vi "Tree Test-1.vi"() -> ()   [LabVIEW 2015]
panel:
  out "Numeric2":i32
  out "Stop 2":bool
  in  "number":i32
  out "Single Selection Display Text":string
  in  "Single Selection Tree":string(tree)="Sine Graph"
  in  "Stop":bool
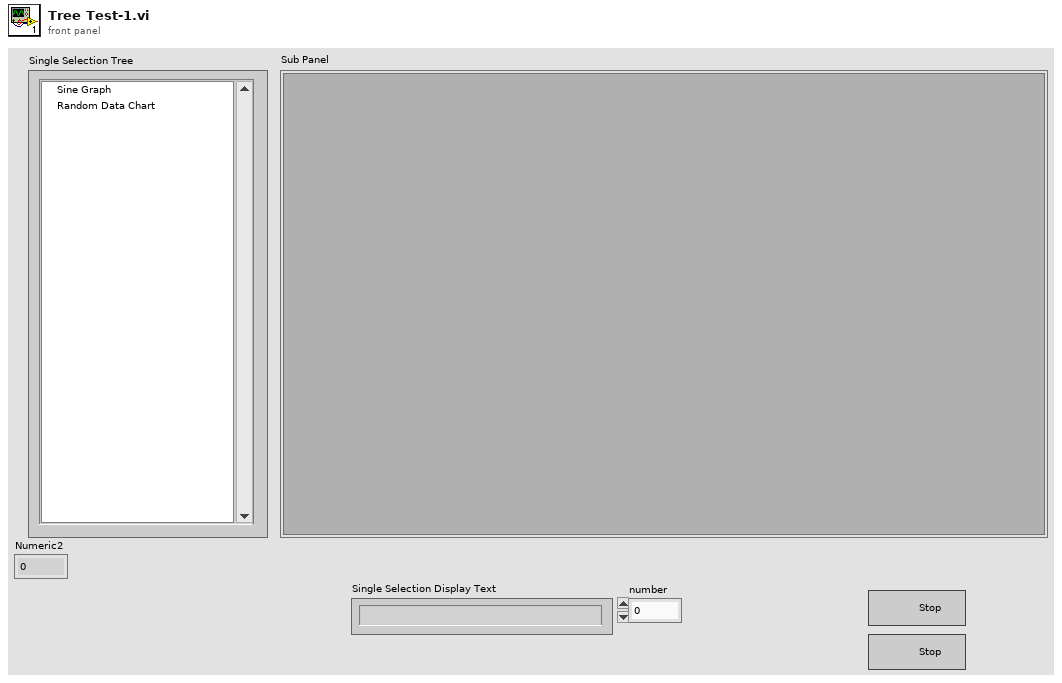
[diagram p1: front panel]
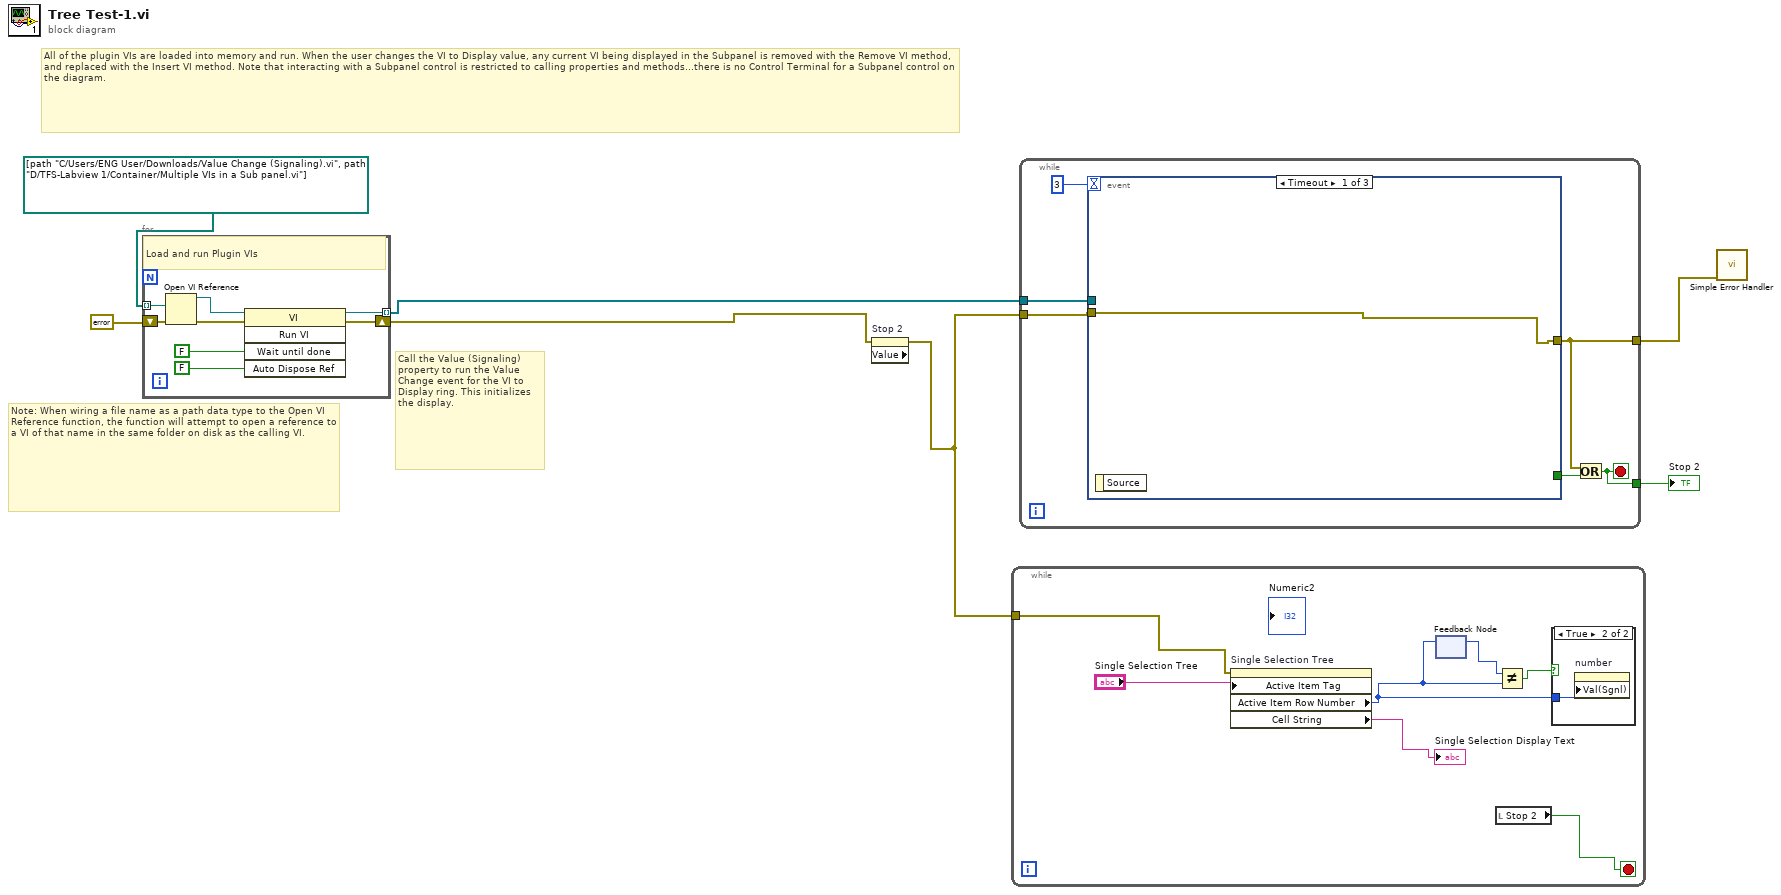
[diagram p0: block diagram]
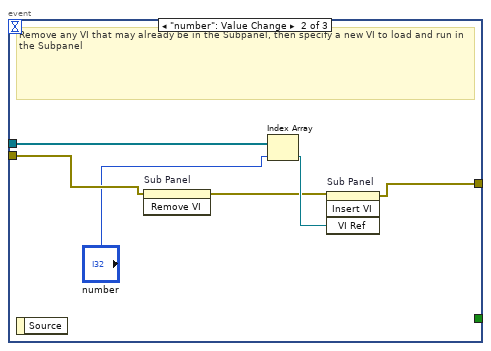
[diagram p3: hidden frame]
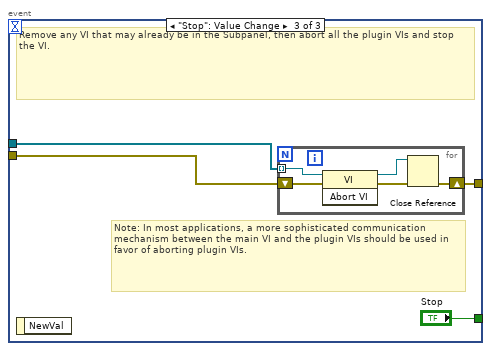
[diagram p4: hidden frame]
diagram:
  # "All of the plugin VIs are loaded into memory and run. When the user changes the VI to Display value, any current VI being displayed in the Subpanel is removed with the Remove VI method, and replaced with the Insert VI method. Note that interacting with a Subpanel control is restricted to calling properties and methods...there is no Control Terminal for a Subpanel control on the diagram."
  # "Note: When wiring a file name as a path data type to the Open VI Reference function, the function will attempt to open a reference to a VI of that name in the same folder on disk as the calling VI."
  # "Call the Value (Signaling) property to run the Value Change event for the VI to Display ring. This initializes the display."
  n1 = for {
    tunnel: path[] [path "C:/Users/ENG User/Downloads/Value Change (Signaling).vi", path "D:/TFS-Labview 1/Container/Multiple VIs in a Sub panel.vi"] -> [w11] mode=indexing
    tunnel: [w10] -> w6 mode=indexing
    shift-right: [w8] -> w2
    shift-left: errorcluster {"status"=FALSE, "code"=0, "source"=""} ("error constant") -> [w9]
    # "Load and run Plugin VIs"
    n2 = Open VI Reference(vi path=w11, error in (no error)=w9) -> (vi reference=w12:refnum<vi>, error out=w13:errorcluster)  [unwired: 4 in]
    n3 = invoke class="VI" method="Run VI"(reference=w12, error in=w13, "Wait until done"=FALSE ("Wait Until Done"), "Auto Dispose Ref"=FALSE ("Auto Dispose Reference")) -> (reference out=w10:refnum<vi>, error out=w8:errorcluster)  [unwired: 1 in, 3 out]
  }
  n4 = property on="Stop 2" class="Bool" props=["Value"](error in=w2) -> (error out=w1:errorcluster)  [unwired: 1 in, 2 out]
  n5 = while {
    tunnel: w1 -> [w19]
    stop <- w20 stop-if-true
    n6 = property on="Single Selection Tree" class="TreeControl (strict)"(error in=w19, "Active Item Tag"="Single Selection Tree") -> ("Active Item Row Number"=w17:i32, "Cell String"=→"Single Selection Display Text":string)  [unwired: 1 in, 2 out]
    n7 = feedback-in #1(w17) -> ()
    n8 = feedback #1() -> (w18:i32)  [unwired: 1 in]
    n9 = local read "Stop 2"() -> (w20:bool)
    n10 = Not Equal?(x=w18, y=w17) -> (x != y?=w16:bool)
    n11 = case shown="True" w16 {
      tunnel: w17 -> [_ w23]
      frame False {
      }
      frame True {
        n12 = property on="number" class="DigNum (strict)"("Val(Sgnl)"=w23) -> ()  [unwired: 2 in, 2 out]
      }
    }
  }
  n13 = while {
    tunnel: [w28] -> w7
    tunnel: w6 -> [w24]
    tunnel: w1 -> [w25]
    tunnel: [w26] -> w3
    stop <- w26 stop-if-true
    n14 = event shown="[0] Timeout" {
      selector: _ -> [_ _ _]
      dyn-events: _ -> [_ _ _]
      timeout: 3 -> [_ _ _]
      tunnel: [_ _ "Stop"] -> w29
      tunnel: [w30 w34 w38] -> w28
      tunnel: w24 -> [_ w36 w39]
      tunnel: w25 -> [w30 w32 w37]
      event Timeout {
        n15 = event-data() -> ()  [unwired: 1 in, 1 out]
      }
      event "number": Value Change {
        # "Remove any VI that may already be in the Subpanel, then specify a new VI to load and run in the Subpanel"
        n16 = event-data() -> ()  [unwired: 1 in, 1 out]
        n17 = invoke on="Sub Panel" class="SubPnl" method="Remove VI"(error in=w32) -> (error out=w33:errorcluster)  [unwired: 2 in, 2 out]
        n18 = Index Array(array=w36, index="number") -> (element=w35:refnum<vi>)
        n19 = invoke on="Sub Panel" class="SubPnl" method="Insert VI"(error in=w33, "VI Ref"=w35) -> (error out=w34:errorcluster)  [unwired: 2 in, 3 out]
      }
      event "Stop": Value Change {
        # "Note: In most applications, a more sophisticated communication mechanism between the main VI and the plugin VIs should be used in favor of aborting plugin VIs."
        # "Remove any VI that may already be in the Subpanel, then abort all the plugin VIs and stop the VI."
        n20 = event-data() -> ()  [unwired: 1 in, 1 out]
        n21 = for {
          shift-right: [w41] -> w38
          shift-left: w37 -> [w45]
          tunnel: w39 -> [w44] mode=indexing
          n22 = invoke class="VI" method="Abort VI"(reference=w44, error in=w45) -> (reference out=w42:refnum<vi>, error out=w43:errorcluster)  [unwired: 1 in, 1 out]
          n23 = Close Reference(reference=w42, error in (no error)=w43) -> (error out=w41:errorcluster)
        }
      }
    }
    n24 = Or(x=w28, y=w29) -> (x .or. y?=w26:bool)
  }
  "Stop 2" <- w3
  n25 = call <vilib>:"Simple Error Handler.vi"("error in (no error)"=w7) -> ()  [unwired: 4 in, 5 out]
